vi "DelayPeriod.vi"(8 "error in (no error)":errorcluster, 11 "TrialBasedExperiment in":refnum<class "WhiteNoiseOrientationDetection.lvclass">) -> (0 "error out":errorcluster, 2 "Timeout":dbl, 3 "TrialBasedExperiment out":refnum<class "WhiteNoiseOrientationDetection.lvclass">)   [LabVIEW 2012, in "WhiteNoiseOrientationDetection.lvclass"]
uses:
  WhiteNoiseOrientationDetection.lvclass
  Trial Based Experiment Statechart/MatlabExperiment/MatlabExperiment.lvclass
  WhiteNoiseOrientationDetection.lvclass/WhiteNoiseOrientationDetection.ctl
  Matlab API/Matlab API.lvlib
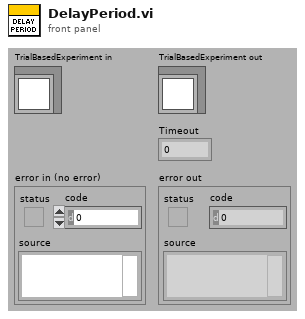
[diagram p1: front panel]
types:
  T1 = cluster{"Intertrial":dbl, "AcquireFixation":dbl, "HoldFixation":dbl, "DelayPeriod":dbl, "ResponsePeriod":dbl}
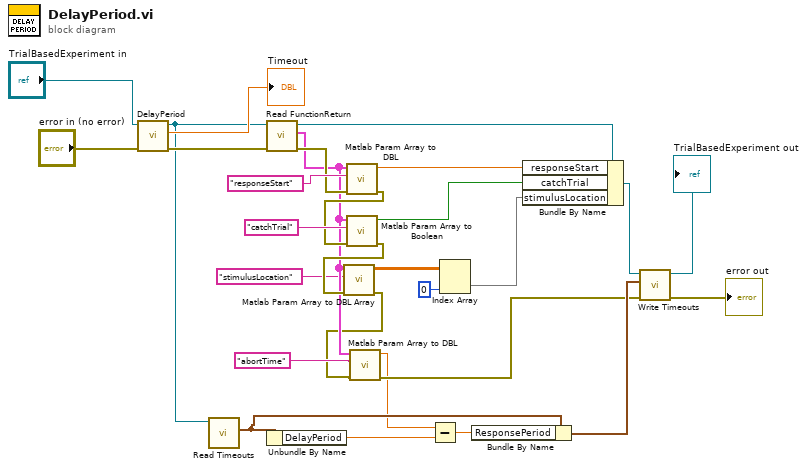
[diagram p0: block diagram]
diagram:
  n1 = call-parent "DelayPeriod.vi"("error in (no error)"="error in (no error)", "TrialBasedExperiment in"="TrialBasedExperiment in") -> ("error out"=w19:errorcluster, "Timeout"=→"Timeout":dbl, "TrialBasedExperiment out"=w18:refnum<class "WhiteNoiseOrientationDetection.lvclass">)  [unwired: 7 in]
  n2 = call-dynamic "Read Timeouts.vi"("TrialBasedExperiment in"=w18) -> ("Timeouts"=w16:T1)  [unwired: 8 in, 2 out]
  n3 = call-dynamic "Read FunctionReturn.vi"("error in (no error)"=w19, "MatlabExperiment in"=w18) -> ("error out"=w23:errorcluster, "FunctionReturn"=w6:cluster{"Name":string, "Data":variant}[], "MatlabExperiment out"=w26:refnum<class "WhiteNoiseOrientationDetection.lvclass">)  [unwired: 7 in]
  n4 = Unbundle By Name(w16) -> ("DelayPeriod"=w8:dbl)
  n5 = call "Matlab Param Array to DBL.vi"("error in (no error)"=w23, "Name"="responseStart", "Matlab Param Array"=w6) -> ("error out"=w22:errorcluster, "data"=w27:dbl)  [unwired: 7 in]
  n6 = call "Matlab Param Array to Boolean.vi"("error in (no error)"=w22, "Name"="catchTrial", "Matlab Param Array"=w6) -> ("error out"=w7:errorcluster, "data"=w25:bool)  [unwired: 7 in]
  n7 = call "Matlab Param Array to DBL Array.vi"("error in (no error)"=w7, "Name"="stimulusLocation", "Matlab Param Array"=w6) -> ("error out"=w4:errorcluster, "data"=w3:dbl[][])  [unwired: 7 in]
  n8 = call "Matlab Param Array to DBL.vi"("error in (no error)"=w4, "Name"="abortTime", "Matlab Param Array"=w6) -> ("error out"=w11:errorcluster, "data"=w9:dbl)  [unwired: 7 in]
  n9 = Subtract(x=w9, y=w8) -> (x-y=w15:dbl)
  n10 = Index Array(array=w3, index (col)=0 ("index (row)")) -> (element=w2:dbl[])  [unwired: 1 in]
  n11 = Bundle By Name(cluster=w16, "ResponsePeriod"=w15) -> (w12:T1)
  n12 = Bundle By Name(cluster=w26, "responseStart"=w27, "catchTrial"=w25, "stimulusLocation"=w2) -> (w14:refnum<class "WhiteNoiseOrientationDetection.lvclass">)
  n13 = call-dynamic "Write Timeouts.vi"("error in (no error)"=w11, "Timeouts"=w12, "TrialBasedExperiment in"=w14) -> ("error out"=→"error out":errorcluster, "TrialBasedExperiment out"=→"TrialBasedExperiment out":refnum<class "WhiteNoiseOrientationDetection.lvclass">)  [unwired: 7 in]
